vi "RotateColorWheel.vi"(11 "SpinnerActions":T1) -> ()   [LabVIEW 2019]
uses:
  Controls/Spinner Actions.ctl
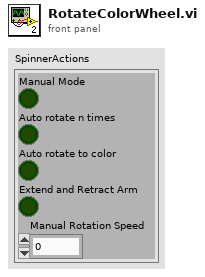
[diagram p1: front panel]
types:
  T1 = typedef "Spinner Actions.ctl" = cluster{"Manual Mode ":bool, "Auto rotate n times":bool, "Auto rotate to color\t":bool, "Extend and Retract Arm\t":bool, "Manual Rotation Speed":dbl}
  T2 = typedef "WPI_MotorControlDeviceRef.ctl" = cluster{"DeviceStatus":errorcluster, "Type":T3, "PWM":cluster{"PWM Channel":T4, "DeadBand":T5}, "CAN":cluster{"Device Number":u8, "SetOutput VI Ref":variant, "GetOutput VI Ref":variant, "Enable VI Ref":variant, "Disable VI Ref":variant, "Data":variant}, "Invert":bool, "DIO PWM":cluster{"PWM \"Enable\" Channel":T4, "DIOChannel":T6, "PWM Rate":dbl}}
  T3 = typedef "WPI_MotorControlType.ctl" = enum16{"PWM", "CAN", "DIO PWM"}
  T4 = typedef "FPGA_DIOPWMChannel.ctl" = enum8{"PWM 0", "PWM 1", "PWM 2", "PWM 3", "PWM 4", "PWM 5", "PWM 6", "PWM 7", "PWM 8", "PWM 9", "PWM MXP 0", "PWM MXP 1", "PWM MXP 2", "PWM MXP 3", "PWM MXP 4", "PWM MXP 5", "PWM MXP 6", "PWM MXP 7", "PWM MXP 8", "PWM MXP 9", "Invalid"}
  T5 = typedef "WPI_PWMDeadband.ctl" = cluster{"Name":string, "maxPositivePwm":i32, "minPositivePwm":i32, "centerPwm":i32, "maxNegativePwm":i32, "minNegativePwm":i32, "angularRange":u16}
  T6 = typedef "FPGA_DIOChannel.ctl" = enum8{"DIO 0", "DIO 1", "DIO 2", "DIO 3", "DIO 4", "DIO 5", "DIO 6", "DIO 7", "DIO 8", "DIO 9", "DIO MXP 0", "DIO MXP 1", "DIO MXP 2", "DIO MXP 3", "DIO MXP 4", "DIO MXP 5", "DIO MXP 6", "DIO MXP 7", "DIO MXP 8", "DIO MXP 9", "DIO MXP 10", "DIO MXP 11", "DIO MXP 12", "DIO MXP 13", "DIO MXP 14", "DIO MXP 15", "SPI Port CS1", "SPI Port CS2", "SPI Port CS3", "SPI Port MISO", "SPI Port MOSI", "Invalid"}
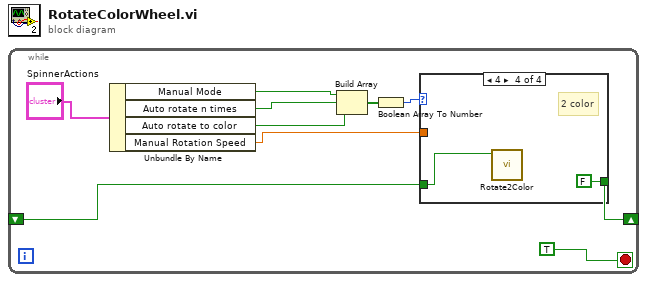
[diagram p0: block diagram]
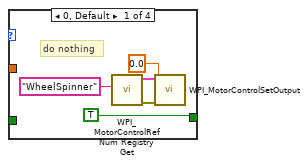
[diagram p2: hidden frame]
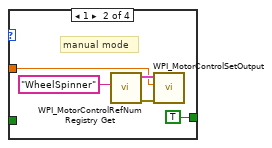
[diagram p3: hidden frame]
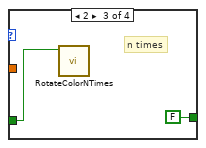
[diagram p4: hidden frame]
diagram:
  n1 = while {
    shift-right: [w7] -> _
    shift-left: _ -> [w6]
    stop <- TRUE stop-if-true
    n2 = Unbundle By Name("SpinnerActions") -> ("Manual Mode"=w5:bool, "Auto rotate n times"=w4:bool, "Auto rotate to color"=w3:bool, "Manual Rotation Speed"=w1:dbl)
    n3 = Build Array(w5, w4, w3) -> (w9:bool[])
    n4 = Boolean Array To Number(Boolean array=w9) -> (number=w10:u32)
    n5 = case shown="4" w10 {
      tunnel: w1 -> [_ w17 _ _]
      tunnel: [TRUE TRUE FALSE FALSE] -> w7
      tunnel: w6 -> [_ _ w22 w24]
      frame 0, Default {
        # "do nothing"
        n6 = call <vilib>:"WPI_MotorControlRefNum Registry Get.vi"("refnum name"="WheelSpinner") -> ("error out"=w15:errorcluster, "MotorControlDevRef"=w14:T2)  [unwired: 9 in]
        n7 = call <vilib>:"WPI_MotorControlSetOutput.vi"("error in (no error)"=w15, "Output"=0.0, "MotorControlDevRef"=w14) -> ()  [unwired: 6 in, 3 out]
      }
      frame 1 {
        # "manual mode"
        n8 = call <vilib>:"WPI_MotorControlRefNum Registry Get.vi"("refnum name"="WheelSpinner") -> ("error out"=w20:errorcluster, "MotorControlDevRef"=w19:T2)  [unwired: 9 in]
        n9 = call <vilib>:"WPI_MotorControlSetOutput.vi"("error in (no error)"=w20, "Output"=w17, "MotorControlDevRef"=w19) -> ()  [unwired: 6 in, 3 out]
      }
      frame 2 {
        # "n times"
        n10 = call "RotateColorNTimes.vi"("Initialize"=w22) -> ()  [unwired: 11 in]
      }
      frame 4 {
        # "2 color"
        n11 = call "Rotate2Color.vi"("Initialize"=w24) -> ()  [unwired: 11 in]
      }
    }
  }
